vi "Launch Nested.vi"(8 "error in (no error)":errorcluster, 11 "Root in":refnum<class "Root.lvclass">) -> (0 "error out":errorcluster, 3 "Root out":refnum<class "Root.lvclass">)   [LabVIEW 2025, in "Root.lvlib" / "Root.lvclass"]
uses:
  Root.lvclass
  Root.lvclass/Root.ctl
  Nested/Nested/Nested.lvclass
  C:/Program Files/National Instruments/LabVIEW 2025/vi.lib/ActorFramework/Actor/Actor.lvclass
  C:/Users/juan_/Desktop/Messages/Nested/Nested/Nested.lvclass
  C:/Users/juan_/Desktop/Messages/Root/Root/Root.lvclass
  <vilib>/ActorFramework/Actor/Actor.lvclass
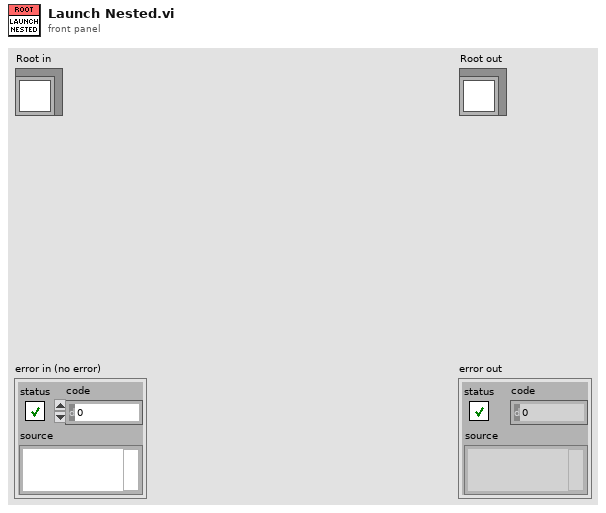
[diagram p1: front panel]
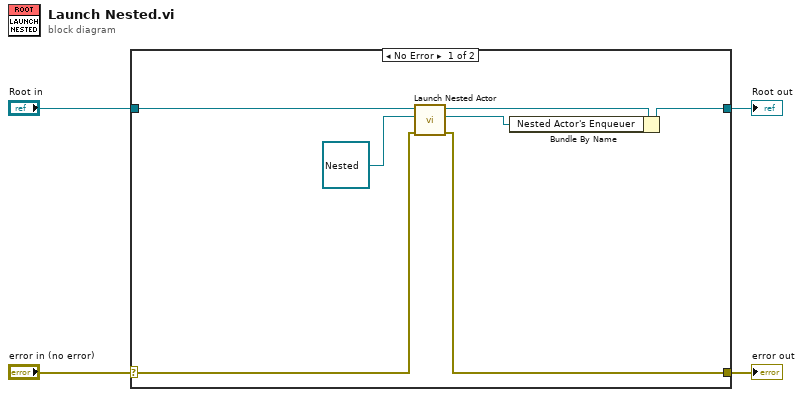
[diagram p0: block diagram]
diagram:
  n1 = case shown="No Error" "error in (no error)" {
    selector: "error in (no error)" -> [w8 w13]
    tunnel: [w7 w13] -> w3
    tunnel: [w6 w12] -> w1
    tunnel: "Root in" -> [w11 w12]
    frame No Error {
      n2 = call <vilib>:"Launch Nested Actor.vi"("error in (no error)"=w8, "Nested Actor"=refnum<class "Nested.lvclass"> refnum ("Nested.lvlib:Nested.lvclass"), "Caller Actor in"=w11) -> ("error out"=w7:errorcluster, "Nested Actor's Enqueuer"=w5:refnum<class "Message Enqueuer.lvclass">, "Caller Actor out"=w10:refnum<class "Root.lvclass">)  [unwired: 6 in]
      n3 = Bundle By Name(cluster=w10, "Nested Actor's Enqueuer"=w5) -> (w6:refnum<class "Root.lvclass">)
    }
    frame Error {
    }
  }
  "error out" <- w3
  "Root out" <- w1
